vi "test_Multiple Global Enum Array Command Messages using Value Change and Trigger with Padding.vi"(8 "error in (no error)":errorcluster, 11 "TestCase in":refnum<class "Instrument Addon System Tests.lvclass">) -> (0 "error out":errorcluster, 3 "TestCase out":refnum<class "Instrument Addon System Tests.lvclass">)   [LabVIEW 2019, in "Instrument Addon System Tests.lvclass"]
uses:
  Instrument Addon System Tests.lvclass
  <vilib>/addons/_JKI Toolkits/VI Tester/TestCase.llb/TestCase.lvclass
  <vilib>/NI VeriStand/Execution/Workspace/NI_VS Workspace ExecutionAPI.lvlib
  <vilib>/NI VeriStand/Execution/Workspace/NI VeriStand - Get Multiple Channel Values.vi
  <vilib>/NI VeriStand/Execution/Workspace/NI VeriStand - Set Multiple Channel Values.vi
  C:/Dev/ni-master/niveristand-custom-device-testing-tools/VeriStandTestCase/VeriStandTestCase.lvclass
  C:/Program Files (x86)/National Instruments/LabVIEW 2019/vi.lib/addons/_JKI Toolkits/VI Tester/TestCase.llb/TestCase.lvclass
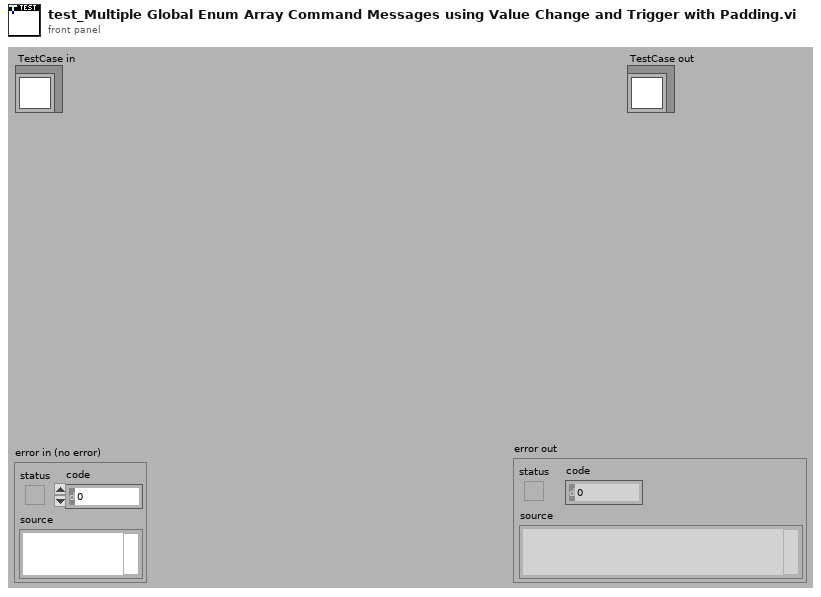
[diagram p1: front panel]
types:
  T1 = typedef "NI_VS Workspace ExecutionAPI.lvlib/WorkspaceAPI.ctl" = refnum<k24>
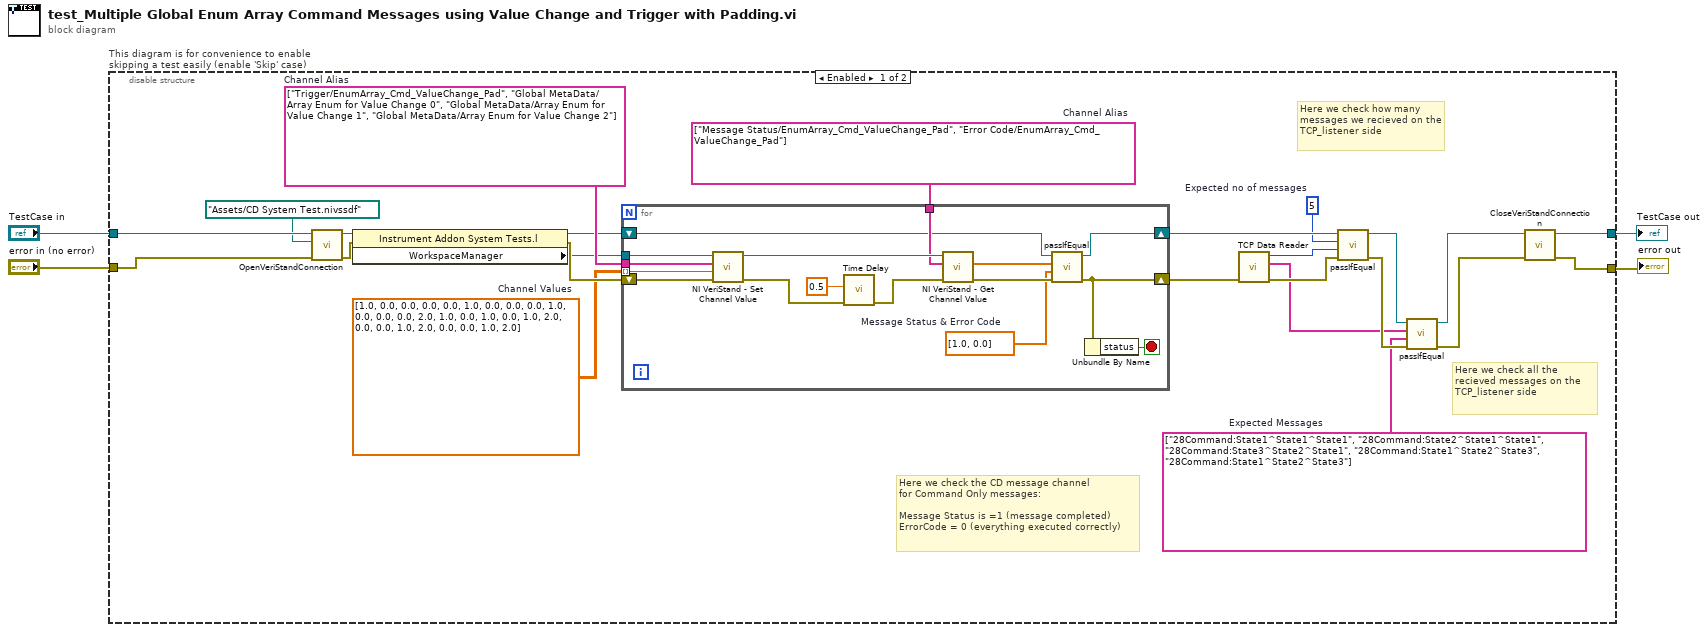
[diagram p0: block diagram]
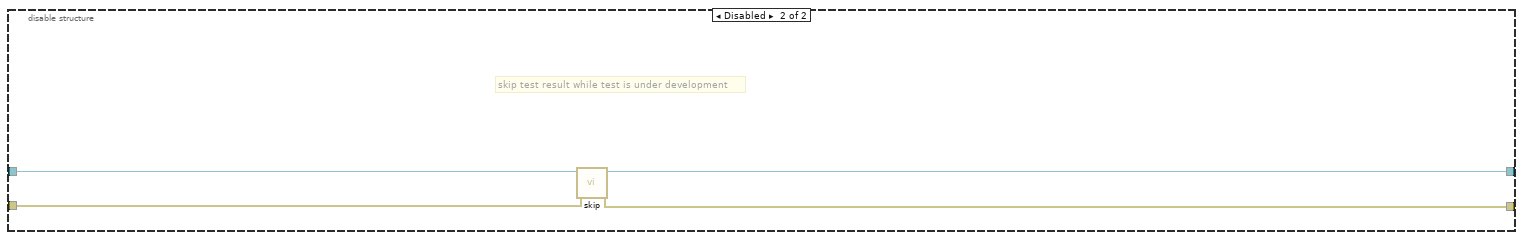
[diagram p2: hidden frame]
diagram:
  n1 = disable-structure "This diagram is for convenience to enable skipping a test easily (enable 'Skip' case)" shown="Enabled" {
    disable-tunnel: "TestCase in" -> [w26 w48]
    disable-tunnel: [w27 w46] -> w1
    disable-tunnel: [w28 w47] -> w3
    disable-tunnel: "error in (no error)" -> [w24 w45]
    frame Enabled {
      w5 = string[] ["28Command:State1^State1^State1", "28Command:State2^State1^State1", "28Command:State3^State2^State1", "28Command:State1^State2^State3", "28Command:State1^State2^State3"]  # Expected Messages
      w8 = 5  # Expected no of messages
      w17 = string[] ["Message Status/EnumArray_Cmd_ValueChange_Pad", "Error Code/EnumArray_Cmd_ValueChange_Pad"]  # Channel Alias
      w19 = dbl[][] [[1.0, 0.0, 0.0, 0.0], [0.0, 1.0, 0.0, 0.0], [0.0, 1.0, 0.0, 0.0], [0.0, 2.0, 1.0, 0.0], [1.0, 0.0, 1.0, 2.0], [0.0, 0.0, 1.0, 2.0], [0.0, 0.0, 1.0, 2.0]]  # Channel Values
      w20 = string[] ["Trigger/EnumArray_Cmd_ValueChange_Pad", "Global MetaData/Array Enum for Value Change 0", "Global MetaData/Array Enum for Value Change 1", "Global MetaData/Array Enum for Value Change 2"]  # Channel Alias
      # "Here we check how many messages we recieved on the TCP_listener side"
      # "Here we check all the recieved messages on the TCP_listener side"
      # "Here we check the CD message channel\nfor Command Only messages:\n\nMessage Status is =1 (message completed)\nErrorCode = 0 (everything executed correctly)"
      n2 = call-dynamic "OpenVeriStandConnection.vi"("error in (no error)"=w24, "System Definition File"=path "Assets/CD System Test.nivssdf", "VeriStand Test Case in"=w26) -> ("error out"=w23:errorcluster, "VeriStand Test Case out"=w25:refnum<class "Instrument Addon System Tests.lvclass">)  [unwired: 6 in, 1 out]
      n3 = property class="Instrument Addon System Tests.l"(reference=w25, error in=w23) -> (reference out=w18:refnum<class "Instrument Addon System Tests.lvclass">, error out=w21:errorcluster, "WorkspaceManager"=w16:T1)
      n4 = for {
        tunnel: w16 -> [w44]
        tunnel: w20 -> [w42]
        tunnel: w19 -> [w30] mode=indexing
        shift-right: [w32] -> w7
        shift-left: w21 -> [w43]
        tunnel: w17 -> [w40]
        shift-right: [w35] -> w15
        shift-left: w18 -> [w36]
        stop <- w31 stop-if-true
        w29 = dbl[] [1.0, 0.0]  # Message Status & Error Code
        n5 = call-poly <vilib>:"NI VeriStand - Set Channel Value.vi"("error in (no error)"=w43, "Values"=w30, "Channels"=w42, "WorkspaceManager in"=w44) -> ("error out"=w38:errorcluster, "WorkspaceManager out"=w41:T1)  [unwired: 6 in]
        n6 = call "Time Delay"("error in (no error)"=w38, "Delay Time (s)"=0.5) -> ("error out"=w37:errorcluster)  [unwired: 9 in]
        n7 = call-poly <vilib>:"NI VeriStand - Get Channel Value.vi"("error in (no error)"=w37, "Channels"=w40, "WorkspaceManager in"=w41) -> ("error out"=w34:errorcluster, "Values"=w33:dbl[])  [unwired: 6 in, 1 out]
        n8 = call-dynamic "passIfEqual.vi"("error in (no error)"=w34, "y"=w29, "x"=w33, "TestCase in"=w36) -> ("error out"=w32:errorcluster, "TestCase out"=w35:refnum<class "Instrument Addon System Tests.lvclass">)  [unwired: 6 in]
        n9 = Unbundle By Name(w32) -> ("status"=w31:bool)
      }
      n10 = call "TCP Data Reader.vi"("error in (no error)"=w7) -> ("error out"=w13:errorcluster, "Recieved Messages"=w6:string[], "No of messages"=w9:i32)  [unwired: 8 in]
      n11 = call-dynamic "passIfEqual.vi"("error in (no error)"=w13, "y"=w9, "x"=w8, "TestCase in"=w15) -> ("error out"=w11:errorcluster, "TestCase out"=w14:refnum<class "Instrument Addon System Tests.lvclass">)  [unwired: 6 in]
      n12 = call-dynamic "passIfEqual.vi"("error in (no error)"=w11, "y"=w5, "x"=w6, "TestCase in"=w14) -> ("error out"=w10:errorcluster, "TestCase out"=w12:refnum<class "Instrument Addon System Tests.lvclass">)  [unwired: 6 in]
      n13 = call-dynamic "CloseVeriStandConnection.vi"("error in (no error)"=w10, "VeriStand Test Case in"=w12) -> ("error out"=w28:errorcluster, "VeriStand Test Case out"=w27:refnum<class "Instrument Addon System Tests.lvclass">)  [unwired: 8 in]
    }
    frame Disabled {
      # "skip test result while test is under development"
      n14 = call <vilib>:"skip.vi"("error in (no error)"=w45, "TestCase in"=w48) -> ("error out"=w47:errorcluster, "TestCase in"=w46:refnum<class "Instrument Addon System Tests.lvclass">)  [unwired: 8 in]
    }
  }
  "error out" <- w3
  "TestCase out" <- w1
